vi "LoopStopTest.vi"(8 "ErrorArray":errorcluster[](array[cluster]), 10 "LoopStopCondition":variant, 11 "Test.lvclass":refnum<class "Test.lvclass">) -> (0 "ErrorArray":errorcluster[](array[cluster]), 2 "StopLoop?":bool, 3 "Test.lvclass":refnum<class "Test.lvclass">)   [LabVIEW 2018, in "Test.lvclass"]
uses:
  Test.lvclass
  Test.lvclass/Test.ctl
  Accessors/Read ErrorSeverity.vi
  Accessors/Read LoopStopCondition.vi
  <vilib>/Utility/error.llb/Error Cluster From Error Code.vi
  <vilib>/ErrorRing/Error Ring.xnode
  <userlib>/NIST/NISTErrorLib/NISTErrorLib.lvlib
panel:
  out "time stamp":timestamp
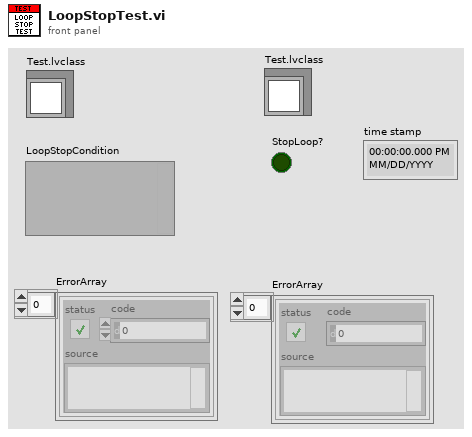
[diagram p1: front panel]
types:
  T1 = typedef "Test.lvclass/LoopStopCondition.ctl" = cluster{"Name":string, "StopCondition":variant}
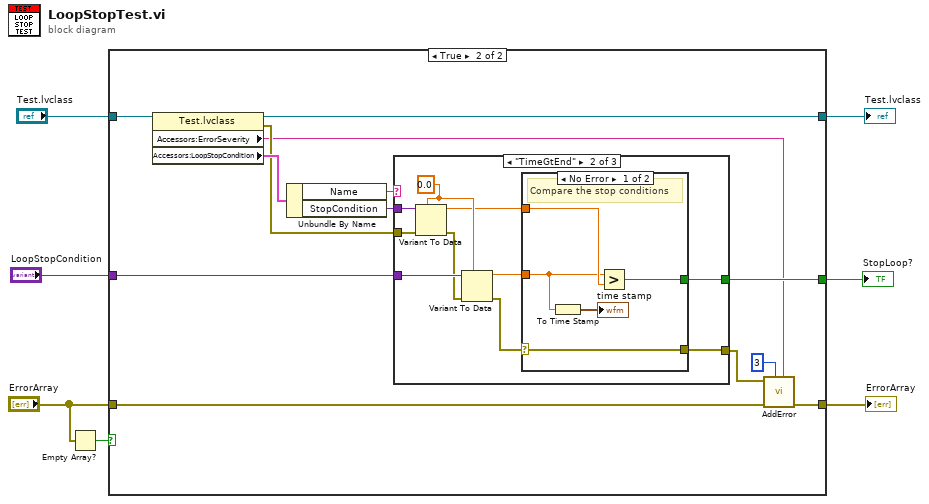
[diagram p0: block diagram]
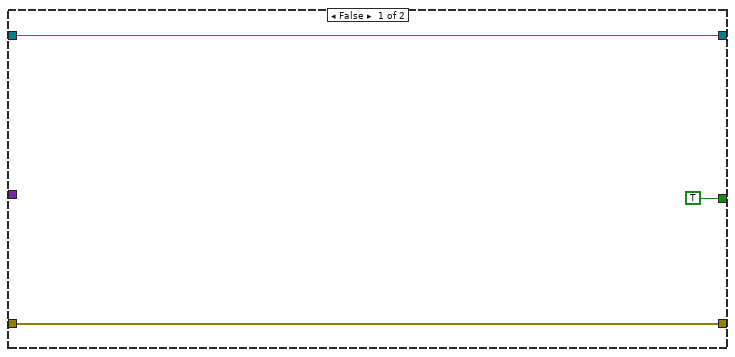
[diagram p2: hidden frame]
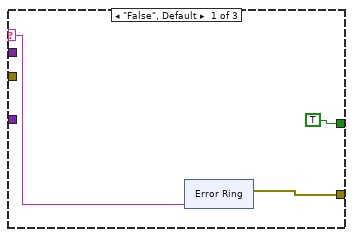
[diagram p3: hidden frame]
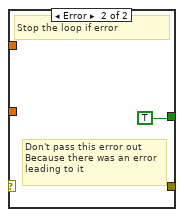
[diagram p4: hidden frame]
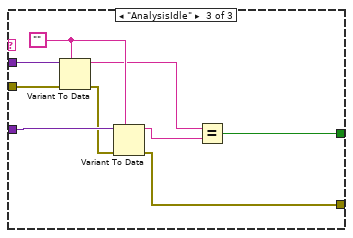
[diagram p5: hidden frame]
diagram:
  n1 = Empty Array?(array="ErrorArray") -> (empty?=w1:bool)
  n2 = case shown="True" w1 {
    tunnel: "Test.lvclass" -> [w9 w23]
    tunnel: "LoopStopCondition" -> [_ w21]
    tunnel: [TRUE w18] -> w5
    tunnel: [w9 w17] -> w4
    tunnel: "ErrorArray" -> [w10 w15]
    tunnel: [w10 w11] -> w3
    frame False {
    }
    frame True {
      n3 = property class="Test.lvclass"(reference=w23) -> (reference out=w17:refnum<class "Test.lvclass">, error out=w16:errorcluster, "Accessors:ErrorSeverity"=w14:string, "Accessors:LoopStopCondition"=w20:T1)  [unwired: 1 in]
      n4 = Unbundle By Name(w20) -> ("Name"=w22:string, "StopCondition"=w19:variant)
      n5 = case shown="\"TimeGtEnd\"" w22 {
        selector: w22 -> [w25 _ _]
        tunnel: w21 -> [_ w43 w57]
        tunnel: w19 -> [_ w42 w58]
        tunnel: [TRUE w37 w51] -> w18
        tunnel: [w26 w34 w50] -> w12
        tunnel: w16 -> [_ w36 w56]
        frame "False", Default {
          n6 = xnode "Error Ring"("parameter 0"=w25) -> ("error out"=w26:errorcluster)
        }
        frame "TimeGtEnd" {
          w41 = 0.0
          n7 = Variant To Data(error in=w36, type=w41, Variant=w42) -> (data=w38:dbl, error out=w40:errorcluster)
          n8 = Variant To Data(error in=w40, type=w41, Variant=w43) -> (data=w39:dbl, error out=w35:errorcluster)
          n9 = case shown="No Error" w35 {
            selector: w35 -> [w46 _]
            tunnel: w39 -> [w45 _]
            tunnel: w38 -> [w48 _]
            tunnel: [w47 TRUE] -> w37
            tunnel: [w46 _] -> w34
            frame No Error {
              # "Compare the stop conditions"
              n10 = To Time Stamp(1:w45) -> (0:→"time stamp":timestamp)
              n11 = Greater?(x=w45, y=w48) -> (0:w47:bool)
            }
            frame Error {
              # "Don't pass this error out\nBecause there was an error\nleading to it"
              # "Stop the loop if error"
            }
          }
        }
        frame "AnalysisIdle" {
          w54 = ""
          n12 = Variant To Data(error in=w56, type=w54, Variant=w58) -> (data=w52:string, error out=w55:errorcluster)
          n13 = Variant To Data(error in=w55, type=w54, Variant=w57) -> (data=w53:string, error out=w50:errorcluster)
          n14 = Equal?(x=w52, y=w53) -> (x = y?=w51:bool)
        }
      }
      n15 = call <userlib>:"AddError.vi"("Severity"=w14, "Priority"=u8 3, "ErrorArray"=w15, "error in (no error)"=w12) -> ("ErrorArray"=w11:errorcluster[])  [unwired: 6 in, 1 out]
    }
  }
  "Test.lvclass" <- w4
  "ErrorArray" <- w3
  "StopLoop?" <- w5
